vi "MagEncoder_cal_v3.vi"() -> ()   [LabVIEW 2014]
uses:
  <vilib>/rvi/FXPMathLib/FxpSinAndCos/subVIs/nifxpmath_SinAndCos_SimConfig.ctl
  <vilib>/rvi/Emulation/niFpgaGetClockAttributes.vi
  <vilib>/rvi/Emulation/niFpgaSctlEmulationGetInTimedLoop.vi
  <vilib>/rvi/Emulation/niFpgaEmulationReportErrorSimple.vi
  <vilib>/rvi/Emulation/niFpgaProcessEmulError.vi
  <vilib>/rvi/interface/RandomDataEmulation/nirviRandomDataMultiElementFPGAFIFO.vi
  <instcachedir>/0/nirviRandomDataMultiElementFPGAFIFO_AD0CFC12EF974623A9C2E4184BC062B2.lvgen/nirviRandomDataMultiElementFPGAFIFO_AD0CFC12EF974623A9C2E4184BC062B2_025.vi
  <vilib>/rvi/interface/RandomDataEmulation/niFpgaRandomDataHandleErrors.vi
  <vilib>/rvi/Emulation/niFpgaCriticalErrorInLSC.vi
  <vilib>/rvi/FXPMathLib/FxpSinAndCos/simVIs/DllFxpSinAndCosTemp_sub.vi
  <vilib>/rvi/eio/common/nirviEmuTemplateMethod_errors.vi
  <vilib>/rvi/DataTransferAndStorage/Container/XNode/niFpgaContainer.xnode
  <vilib>/rvi/interface/RandomDataEmulation/nirviRandomDataFpgaMultiElementTemplate.vi
  <vilib>/rvi/FXPMathLib/FxpSinAndCos/XNode/nifxpmath_SinAndCos.xnode
  <vilib>/eio/EIONode/EIONode.xnode
  <vilib>/rvi/Analysis/measure/butterworth/XNode/niFpgaButterworthFilter.xnode
panel:
  in  "Vy (mm/s)":fxp<+/-,30,6>
  out "Dyr_ramp":fxp<+/-,32,7>
  in  "Dyr_stroke":fxp<+/-,32,7>
  out "Dpr_ramp":fxp<+/-,32,7>
  in  "Dpr_stroke":fxp<+/-,32,7>
  in  "Vp (mm/s)":fxp<+/-,30,6>
  out "omega_p (Mavg w. f)":fxp<+/-,36,18>
  in  "scaled coefficients":i32[](array[numeric])=[946630756, 63555534]
  in  "FIFO":i16(ring) items=["Pitch_F+P", "Yaw_F+P"]
  out "PID (kHz)":fxp<+/-,20,10>
  out "Dy1_d (T)":fxp<+/-,36,13>
  out "omega_y1 (T)":fxp<+/-,36,13>
  out "Dp1_d (T)":fxp<+/-,36,13>
  out "omega_p1 (T)":fxp<+/-,36,13>
  out "Dy2_d (T)":fxp<+/-,36,13>
  out "Dp2_d (T)":fxp<+/-,36,13>
  out "omega_y2 (T)":fxp<+/-,36,13>
  out "omega_p2 (T)":fxp<+/-,36,13>
  out "mt_omega_y2":u32
  out "mt_omega_p2":u32
  out "rad_y2":fxp<+/-,33,20>
  out "D_y2":fxp<+/-,32,7>
  out "rad_y1":fxp<+/-,33,20>
  out "D_y1":fxp<+/-,32,7>
  out "Encoder Position_y1":i32
  out "Encoder Position_y2":i32
  out "Encoder Position_p2":i32
  out "D_p2":fxp<+/-,32,7>
  out "rad_p2":fxp<+/-,33,20>
  out "D_p1":fxp<+/-,32,7>
  out "rad_p1":fxp<+/-,33,20>
  out "Encoder Position_p1":i32
  in  "Mag. factor_y":fxp<+/-,20,3>
  in  "Mag. encoder_y":bool
  out "omega_y (rad/s)":fxp<+/-,36,13>
  out "Dy_d (mm/s)":fxp<+/-,36,13>
  in  "Vy. Est.":i16(ring) items=["T", "Mavg"]
  out "omega_y (Mavg)":fxp<+/-,36,14>
  out "Dy_d (Mavg)":fxp<+/-,36,14>
  in  "Dy_d_M_avg_Tc (uSec)":i32
  out "Dp_d (Mavg)":fxp<+/-,36,14>
  out "omega_p (Mavg)":fxp<+/-,36,14>
  in  "Dp_d_M_avg_Tc (uSec)":i32
  out "Dp_d (T)":fxp<+/-,36,13>
  out "omega_p (T)":fxp<+/-,36,13>
  in  "Vp. Est.":i16(ring) items=["T", "Mavg"]
  in  "Mag. factor_p":fxp<+/-,20,3>
  in  "Mag. encoder_p":bool
  in  "Belt_out_p":fxp<+/-,7,7>
  in  "Belt_in_p":fxp<+/-,6,6>
  in  "Belt_out_y":fxp<+/-,7,7>
  in  "Belt_in_y":fxp<+/-,6,6>
  in  "mt0_omega_p":u32
  in  "Encoder reset":bool
  out "Dpr_sin":fxp<+/-,32,7>
  in  "Sin offset_p":fxp<+/-,22,7>
  in  "Sin magnitude_p":fxp<+/-,21,6>
  in  "Sin wave freq._p (Hz)":fxp<+/-,32,6>
  in  "Dpr_step":fxp<+/-,32,7>
  out "Dpr_for":fxp<+/-,32,7>
  in  "Command_p":i16(ring) items=["Step", "Sine", "Ramp"]
  out "Fp_PID":fxp<+/-,36,16>
  in  "Kp_p":fxp<+/-,32,13>
  out "va_p":fxp<+/-,36,7>
  out "vb_p":fxp<+/-,37,8>
  out "vq_p_F":fxp<+/-,20,5> format="%.57g"
  out "vd_p_F":fxp<+/-,20,5>
  in  "Stop motor_p":bool
  out "Dp_d (mm/s)":fxp<+/-,36,13>
  out "omega_p (rad/s)":fxp<+/-,36,13>
  out "mt_omega_p1":u32
  out "rad_p(NrTheta)":fxp<+/-,33,20>
  out "D_p(mm)":fxp<+/-,32,7>
  out "Encoder Position_p":i32
  in  "Encoder reset_p":bool
  out "Dyr_for":fxp<+/-,32,7>
  in  "Command_y":i16(ring) items=["Step", "Sine", "Ramp"]
  out "vb_y":fxp<+/-,38,8>
  out "va_y":fxp<+/-,38,8>
  out "Dyr_sin":fxp<+/-,32,7>
  in  "Sin offset_y":fxp<+/-,22,7>
  in  "Sin magnitude_y":fxp<+/-,21,6>
  out "Time now(s)":fxp<+,52,14>
  in  "Sin wave freq._y (Hz)":fxp<+/-,32,6>
  in  "Dyr_step":fxp<+/-,32,7>
  out "Fy_PID":fxp<+/-,36,16>
  in  "Kp_y":fxp<+/-,32,13>
  out "vq_y_F":fxp<+/-,20,5> format="%.57g"
  out "vd_y_F":fxp<+/-,20,5>
  in  "Stop motor_y":bool
  out "Dy_d (T)":fxp<+/-,36,13>
  out "omega_y (T)":fxp<+/-,36,13>
  in  "mt0_omega_y":u32
  out "mt_omega_y1":u32
  out "rad_y(NrTheta)":fxp<+/-,33,20>
  out "D_y(mm)":fxp<+/-,32,7>
  out "Encoder Position_y":i32
  in  "Encoder reset_y":bool
  in  "Ini coe.":bool
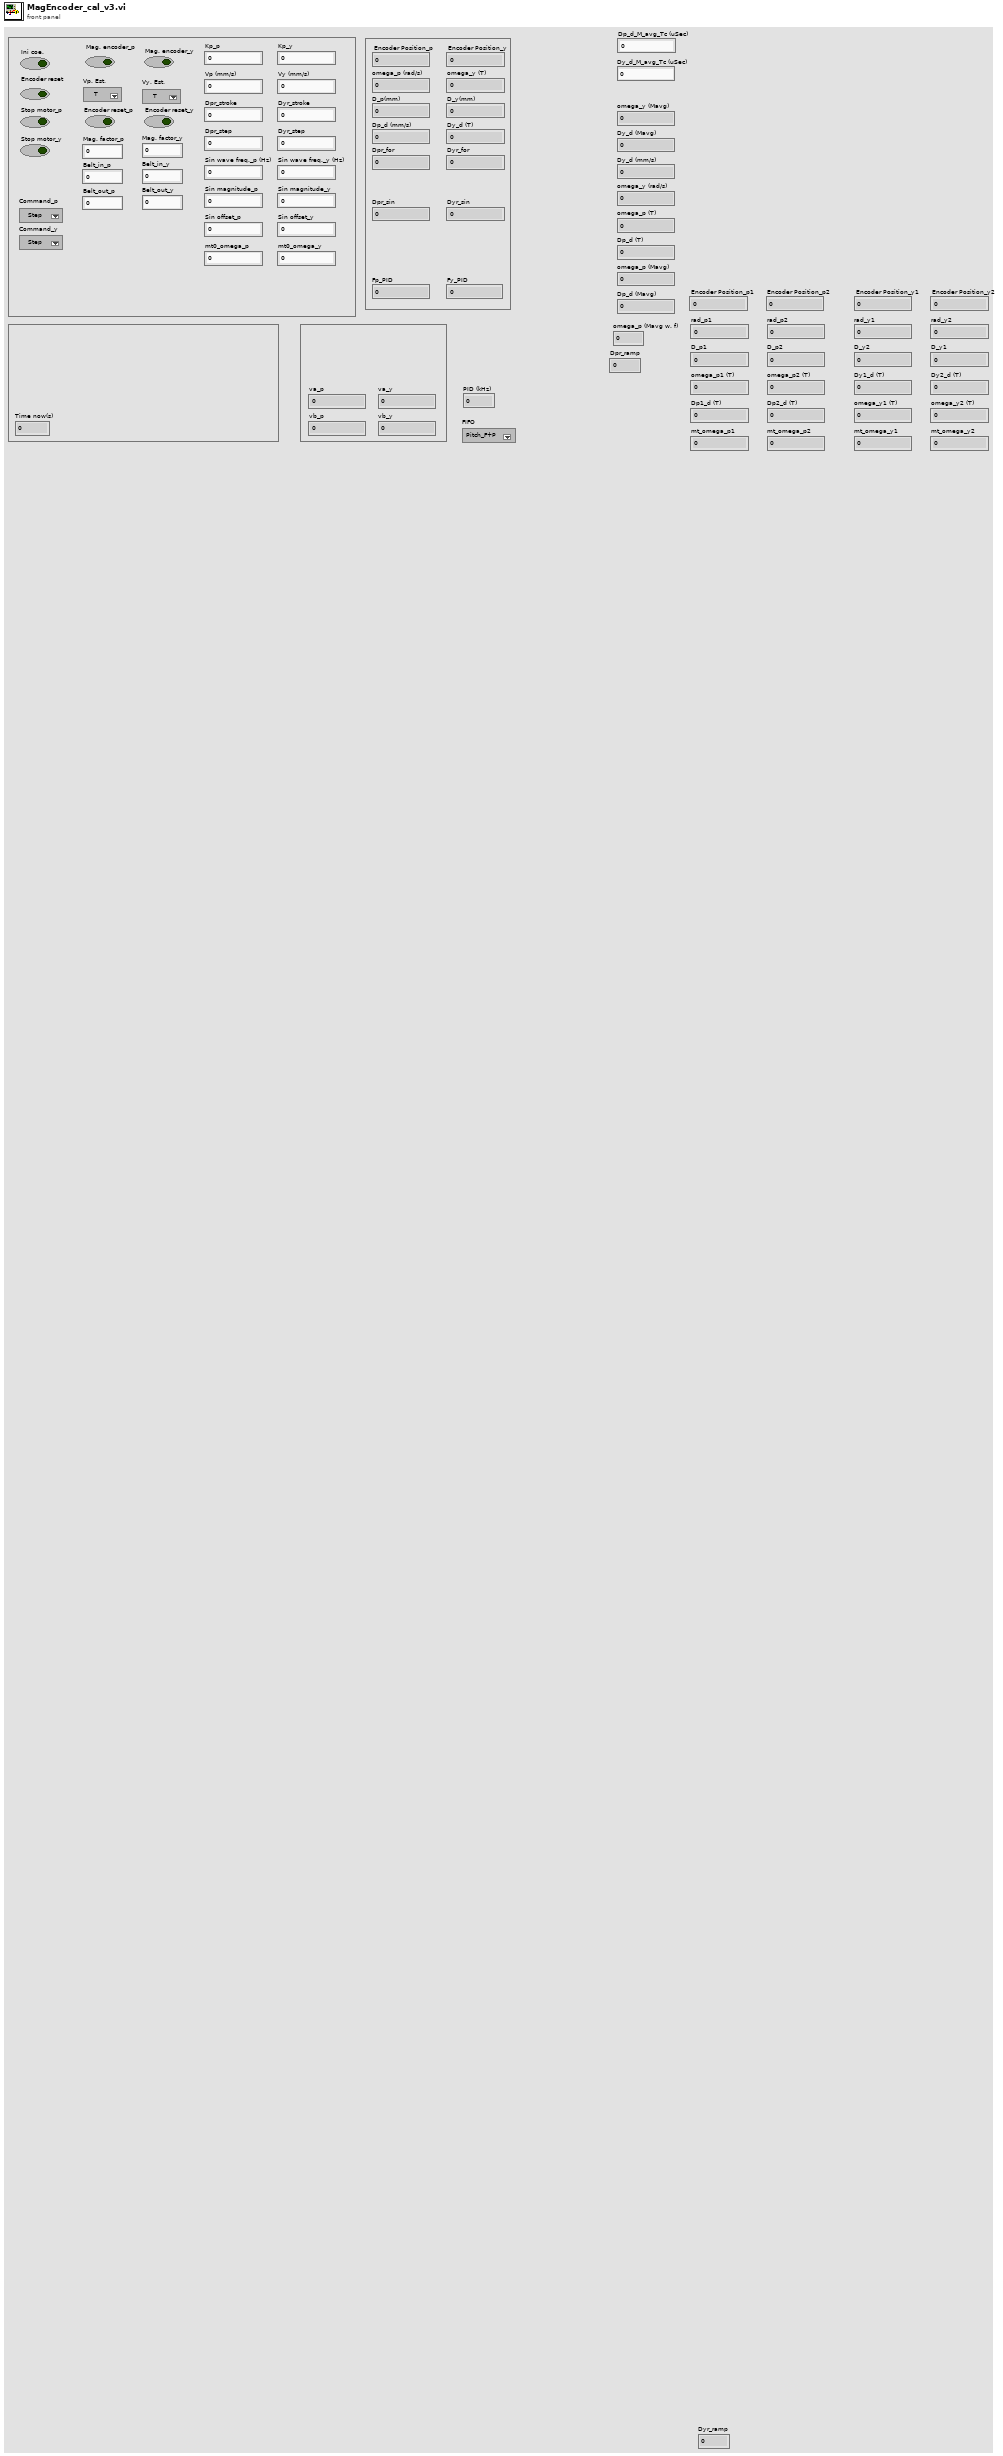
[diagram p1: front panel]
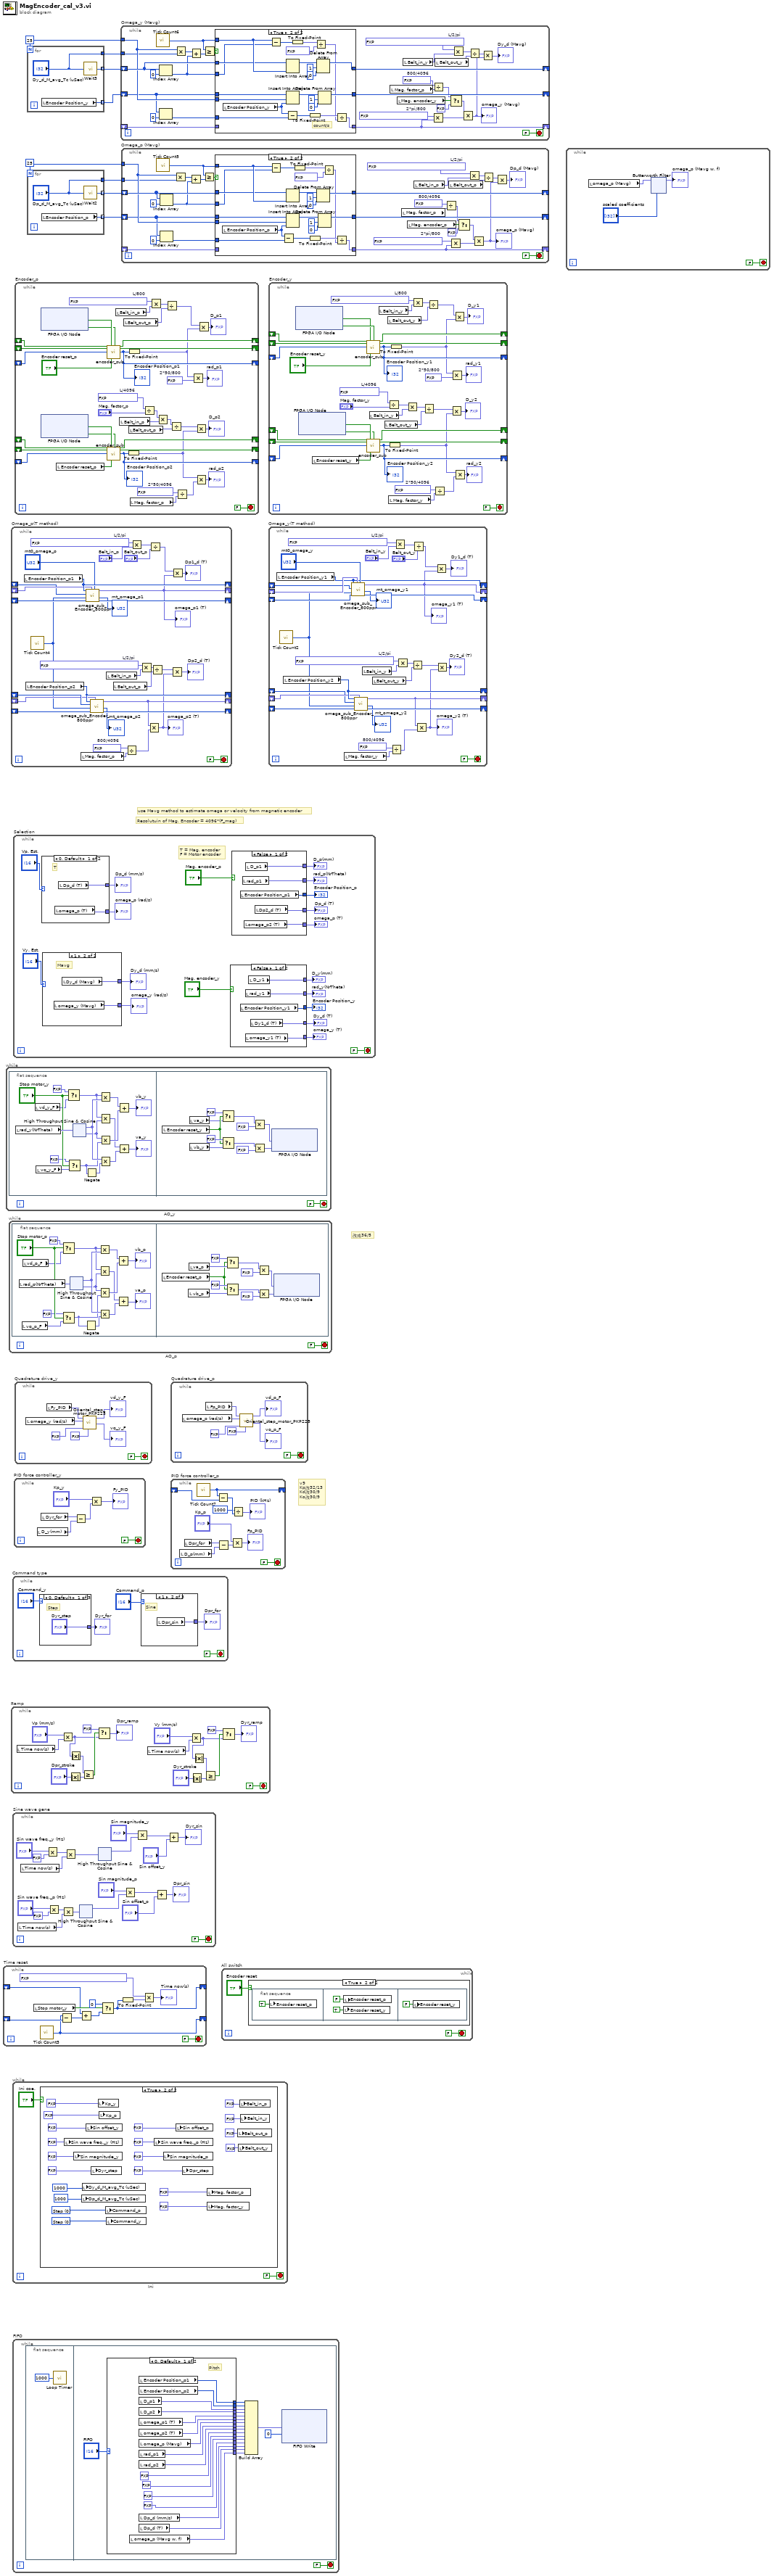
[diagram p0: block diagram]
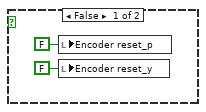
[diagram p4: hidden frame]
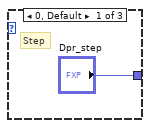
[diagram p5: hidden frame]
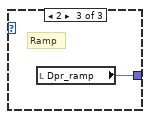
[diagram p6: hidden frame]
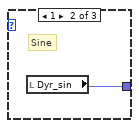
[diagram p7: hidden frame]
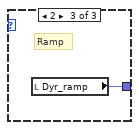
[diagram p8: hidden frame]
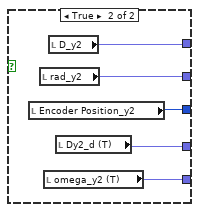
[diagram p9: hidden frame]
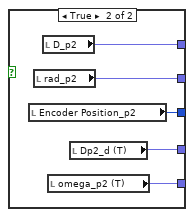
[diagram p10: hidden frame]
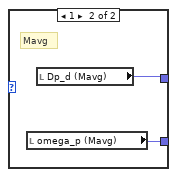
[diagram p11: hidden frame]
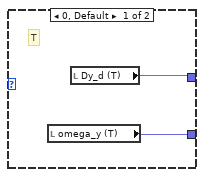
[diagram p12: hidden frame]
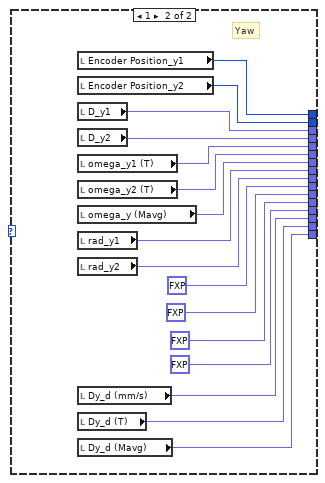
[diagram p14: hidden frame]
diagram:
  w5 = 25
  w8 = 25
  # "改成36/5"
  # "v9\nKp改32/13\nKd改30/9\nKo改30/9"
  # "Resolutuin of Mag. Encoder = 4096*(F_mag)"
  # "use Mavg method to estimate omega or velocity from magnetic encoder"
  n1 = while "Time reset" {
    shift-right: [w18] -> _
    shift-left: _ -> [w19]
    shift-right: [w13] -> _
    shift-left: _ -> [w14]
    stop <- FALSE stop-if-true
    n2 = local read "Stop motor_y"() -> (w20:bool)
    n3 = call "Tick Count3"() -> ("Tick Count(uSec)"=w18:u32)
    n4 = Subtract(x=w18, y=w19) -> (x-y=w17:u32)
    n5 = Add(x=w14, y=w17) -> (x+y=w16:u32)
    n6 = Select(t=u32 0, s=w20, f=w16) -> (s? t:f=w13:u32)
    n7 = To Fixed-Point(number=w13) -> (fixed-point=w12:fxp<+,32,32>)  [unwired: 1 in]
    n8 = Multiply(x=fxp<+,20,-18> 1.0000003385357559e-06, y=w12) -> (x*y=→"Time now(s)":fxp<+,52,14>)
  }
  n9 = while "AO_y" {
    stop <- FALSE stop-if-true
    n10 = flat-sequence {
      frame #0 {
        n11 = local read "rad_y(NrTheta)"() -> (w38:fxp<+/-,33,20>)
        n12 = local read "vd_y_F"() -> (w36:fxp<+/-,20,5>)
        n13 = local read "vq_y_F"() -> (w35:fxp<+/-,20,5>)
        n14 = Select(t=fxp<+/-,20,5> 0.0, s="Stop motor_y", f=w36) -> (s? t:f=w30:fxp<+/-,20,5>)
        n15 = Select(t=fxp<+/-,20,5> 0.0, s="Stop motor_y", f=w35) -> (s? t:f=w29:fxp<+/-,20,5>)
        n16 = xnode "High Throughput Sine & Cosine"("x (pi)"=w38) -> ("sin(x)"=w32:fxp<+/-,17,2>, "cos(x)"=w31:fxp<+/-,17,2>)
        n17 = Negate(x=w29) -> (-x=w28:fxp<+/-,21,6>)
        n18 = Multiply(x=w30, y=w32) -> (x*y=w27:fxp<+/-,37,7>)
        n19 = Multiply(x=w30, y=w31) -> (x*y=w25:fxp<+/-,37,7>)
        n20 = Multiply(x=w31, y=w29) -> (x*y=w26:fxp<+/-,37,7>)
        n21 = Multiply(x=w32, y=w28) -> (x*y=w24:fxp<+/-,36,6>)
        n22 = Add(x=w27, y=w26) -> (x+y=→"vb_y":fxp<+/-,38,8>)
        n23 = Add(x=w25, y=w24) -> (x+y=→"va_y":fxp<+/-,37,7>)
      }
      frame #1 {
        n24 = local read "Encoder reset_y"() -> (w71:bool)
        n25 = local read "va_y"() -> (w70:fxp<+/-,38,8>)
        n26 = local read "vb_y"() -> (w69:fxp<+/-,38,8>)
        n27 = Select(t=fxp<+,2,2> 3.0, s=w71, f=w70) -> (s? t:f=w75:fxp<+/-,38,8>)
        n28 = Select(t=fxp<+,1,1> 0.0, s=w71, f=w69) -> (s? t:f=w74:fxp<+/-,38,8>)
        n29 = Multiply(x=w75, y=fxp<+/-,1,0> -0.5) -> (x*y=w78:fxp<+/-,36,6>)
        n30 = Multiply(x=w74, y=fxp<+/-,1,0> -0.5) -> (x*y=w79:fxp<+/-,36,5>)
        n31 = xnode "FPGA I/O Node"("Mod8/AO2"=w78, "Mod8/AO3"=w79) -> ()  [unwired: 2 in, 2 out]
      }
    }
  }
  n32 = while "AO_p" {
    stop <- FALSE stop-if-true
    n33 = flat-sequence {
      frame #0 {
        n34 = local read "rad_p(NrTheta)"() -> (w92:fxp<+/-,33,20>)
        n35 = local read "vq_p_F"() -> (w93:fxp<+/-,20,5>)
        n36 = local read "vd_p_F"() -> (w95:fxp<+/-,20,5>)
        n37 = Select(t=fxp<+/-,20,5> 0.0, s="Stop motor_p", f=w95) -> (s? t:f=w84:fxp<+/-,20,5>)
        n38 = Select(t=fxp<+,1,1> 0.0, s="Stop motor_p", f=w93) -> (s? t:f=w83:fxp<+/-,20,5>)
        n39 = xnode "High Throughput Sine & Cosine"("x (pi)"=w92) -> ("sin(x)"=w86:fxp<+/-,16,2>, "cos(x)"=w85:fxp<+/-,16,2>)
        n40 = Negate(x=w83) -> (-x=w91:fxp<+/-,21,6>)
        n41 = Multiply(x=w84, y=w86) -> (x*y=w90:fxp<+/-,36,7>)
        n42 = Multiply(x=w84, y=w85) -> (x*y=w88:fxp<+/-,36,7>)
        n43 = Multiply(x=w85, y=w83) -> (x*y=w89:fxp<+/-,36,7>)
        n44 = Multiply(x=w86, y=w91) -> (x*y=w87:fxp<+/-,35,6>)
        n45 = Add(x=w90, y=w89) -> (x+y=→"vb_p":fxp<+/-,37,8>)
        n46 = Add(x=w88, y=w87) -> (x+y=→"va_p":fxp<+/-,36,7>)
      }
      frame #1 {
        n47 = local read "Encoder reset_p"() -> (w128:bool)
        n48 = local read "vb_p"() -> (w129:fxp<+/-,37,8>)
        n49 = local read "va_p"() -> (w130:fxp<+/-,36,7>)
        n50 = Select(t=fxp<+,2,2> 3.0, s=w128, f=w130) -> (s? t:f=w136:fxp<+/-,36,7>)
        n51 = Select(t=fxp<+,1,1> 0.0, s=w128, f=w129) -> (s? t:f=w135:fxp<+/-,37,8>)
        n52 = Multiply(x=w136, y=fxp<+/-,1,0> -0.5) -> (x*y=w131:fxp<+/-,36,5>)
        n53 = Multiply(x=w135, y=fxp<+/-,1,0> -0.5) -> (x*y=w132:fxp<+/-,36,5>)
        n54 = xnode "FPGA I/O Node"("Mod8/AO0"=w131, "Mod8/AO1"=w132) -> ()  [unwired: 2 in, 2 out]
      }
    }
  }
  n55 = while "Ramp" {
    stop <- FALSE stop-if-true
    n56 = local read "Time now(s)"() -> (w156:fxp<+,52,14>)
    n57 = Multiply(x="Vp (mm/s)", y=w156) -> (x*y=w143:fxp<+/-,64,20>)
    n58 = Absolute Value(x="Dpr_stroke") -> (abs(x)=w145:fxp<+,32,7>)
    n59 = Absolute Value(x=w143) -> (abs(x)=w144:fxp<+,64,20>)
    n60 = Greater Or Equal?(x=w144, y=w145) -> (x >= y?=w155:bool)
    n61 = Select(t=fxp<+/-,64,46> 0.0, s=w155, f=w143) -> (s? t:f=→"Dpr_ramp":fxp<+/-,64,46>)
    n62 = local read "Time now(s)"() -> (w149:fxp<+,52,14>)
    n63 = Multiply(x="Vy (mm/s)", y=w149) -> (x*y=w139:fxp<+/-,64,20>)
    n64 = Absolute Value(x="Dyr_stroke") -> (abs(x)=w141:fxp<+,32,7>)
    n65 = Absolute Value(x=w139) -> (abs(x)=w140:fxp<+,64,20>)
    n66 = Greater Or Equal?(x=w140, y=w141) -> (x >= y?=w152:bool)
    n67 = Select(t=fxp<+/-,64,46> 0.0, s=w152, f=w139) -> (s? t:f=→"Dyr_ramp":fxp<+/-,64,46>)
  }
  n68 = while "Omega_p(T method)" {
    shift-right: [w190] -> _
    shift-left: _ -> [w188]
    shift-right: [w161] -> _
    shift-left: _ -> [w189]
    shift-right: [w186] -> _
    shift-left: _ -> [w187]
    shift-right: [w177] -> _
    shift-left: _ -> [w176]
    shift-right: [w170] -> _
    shift-left: _ -> [w175]
    shift-right: [w174] -> _
    shift-left: _ -> [w173]
    stop <- FALSE stop-if-true
    w168 = fxp<+/-,32,0> 0.3183098859153688  # L/2/pi
    w179 = fxp<+,32,0> 0.1953125  # 800/4096
    w183 = fxp<+/-,32,0> 0.3183098859153688  # L/2/pi
    n69 = local read "Encoder Position_p1"() -> (w190:i32)
    n70 = local read "Encoder Position_p2"() -> (w177:i32)
    n71 = call "Tick Count4"() -> ("Tick Count(Ticks)"=w172:u32)
    n72 = local read "Mag. factor_p"() -> (w178:fxp<+/-,20,3>)
    n73 = call "omega_sub_Encoder_800ppr.vi"("mt0"="mt0_omega_p", "omega_pre"=w189, "ticks_m_pre"=w187, "ticks"=w172, "count_pre"=w188, "count"=w190) -> ("ticks_m"=w186:u32, "mt"=→"mt_omega_p1":u32, "omega"=w161:fxp<+/-,36,13>)  [unwired: 3 in]
    "omega_p1 (T)" <- w161
    n74 = call "omega_sub_Encoder_800ppr.vi"("omega_pre"=w175, "ticks_m_pre"=w173, "ticks"=w172, "count_pre"=w176, "count"=w177) -> ("ticks_m"=w174:u32, "mt"=→"mt_omega_p2":u32, "omega"=w170:fxp<+/-,36,13>)  [unwired: 4 in]
    n75 = local read "Belt_in_p"() -> (w166:fxp<+/-,6,6>)
    n76 = local read "Belt_out_p"() -> (w165:fxp<+/-,7,7>)
    n77 = Divide(x=w179, y=w178) -> (x/y=w169:fxp<+/-,32,1>)
    n78 = Multiply(x=w183, y="Belt_in_p") -> (x*y=w181:fxp<+/-,38,6>)
    n79 = Multiply(x=w168, y=w166) -> (x*y=w167:fxp<+/-,38,6>)
    n80 = Multiply(x=w170, y=w169) -> (x*y=w159:fxp<+/-,36,13>)
    "omega_p2 (T)" <- w159
    n81 = Divide(x=w181, y="Belt_out_p") -> (x/y=w162:fxp<+/-,20,1>)
    n82 = Divide(x=w167, y=w165) -> (x/y=w160:fxp<+/-,45,6>)
    n83 = Multiply(x=w160, y=w159) -> (x*y=→"Dp2_d (T)":fxp<+/-,36,13>)
    n84 = Multiply(x=w162, y=w161) -> (x*y=→"Dp1_d (T)":fxp<+/-,36,13>)
  }
  n85 = while "Command type" {
    stop <- FALSE stop-if-true
    n86 = case shown="0, Default" "Command_y" {
      tunnel: ["Dyr_step" w200 w201] -> w194
      frame 0, Default {
        # "Step"
      }
      frame 1 {
        # "Sine"
        n87 = local read "Dyr_sin"() -> (w200:fxp<+/-,32,7>)
      }
      frame 2 {
        # "Ramp"
        n88 = local read "Dyr_ramp"() -> (w201:fxp<+/-,32,7>)
      }
    }
    "Dyr_for" <- w194
    n89 = case shown="1" "Command_p" {
      tunnel: ["Dpr_step" w197 w198] -> w192
      frame 0, Default {
        # "Step"
      }
      frame 1 {
        # "Sine"
        n90 = local read "Dpr_sin"() -> (w197:fxp<+/-,32,7>)
      }
      frame 2 {
        # "Ramp"
        n91 = local read "Dpr_ramp"() -> (w198:fxp<+/-,32,7>)
      }
    }
    "Dpr_for" <- w192
  }
  n92 = while "Sine wave gene" {
    stop <- FALSE stop-if-true
    n93 = local read "Time now(s)"() -> (w208:fxp<+,52,14>)
    n94 = local read "Time now(s)"() -> (w219:fxp<+,52,14>)
    n95 = Multiply(x="Sin wave freq._y (Hz)", y=fxp<+/-,10,3> 2.0) -> (x*y=w220:fxp<+/-,41,9>)
    n96 = Multiply(x="Sin wave freq._p (Hz)", y=fxp<+/-,10,3> 2.0) -> (x*y=w212:fxp<+/-,42,9>)
    n97 = Multiply(x=w212, y=w208) -> (x*y=w209:fxp<+/-,41,19>)
    n98 = Multiply(x=w220, y=w219) -> (x*y=w218:fxp<+/-,41,19>)
    n99 = xnode "High Throughput Sine & Cosine"("x (pi)"=w209) -> ("sin(x)"=w203:fxp<+/-,20,2>)  [unwired: 1 out]
    n100 = xnode "High Throughput Sine & Cosine"("x (pi)"=w218) -> ("sin(x)"=w213:fxp<+/-,20,2>)  [unwired: 1 out]
    n101 = Multiply(x="Sin magnitude_p", y=w203) -> (x*y=w206:fxp<+/-,41,8>)
    n102 = Multiply(x="Sin magnitude_y", y=w213) -> (x*y=w216:fxp<+/-,41,8>)
    n103 = Add(x=w206, y="Sin offset_p") -> (x+y=→"Dpr_sin":fxp<+/-,41,8>)
    n104 = Add(x=w216, y="Sin offset_y") -> (x+y=→"Dyr_sin":fxp<+/-,41,8>)
  }
  n105 = while "Ini" {
    stop <- FALSE stop-if-true
    n106 = case shown="True" "Ini coe." {
      frame False {
      }
      frame True {
        w298 = i16 0 items=["Step", "Sine"] ("Command_p")
        w299 = i16 0 items=["Step", "Sine"] ("Command_y")
        n107 = local write "Sin wave freq._y (Hz)"(fxp<+/-,32,6> 1.0 ("Sin wave freq. (Hz)")) -> ()
        n108 = local write "Sin magnitude_y"(fxp<+/-,22,7> 5.0 ("Sin magnitude")) -> ()
        n109 = local write "Dp_d_M_avg_Tc (uSec)"(u32 1000 ("D_d_M_avg_Tc (uSec)")) -> ()
        n110 = local write "Dy_d_M_avg_Tc (uSec)"(1000 ("Dy_d_M_avg_Tc (uSec)")) -> ()
        n111 = local write "Sin offset_y"(fxp<+/-,38,9> 0.0 ("Sin offset")) -> ()
        n112 = local write "Dyr_step"(fxp<+/-,22,7> 0.0 ("Dr")) -> ()
        n113 = local write "Kp_y"(fxp<+/-,36,9> 30.0 ("Kp")) -> ()
        n114 = local write "Kp_p"(fxp<+/-,36,9> 30.0 ("Kp_p")) -> ()
        n115 = local write "Command_p"(w298) -> ()
        n116 = local write "Command_y"(w299) -> ()
        n117 = local write "Sin wave freq._p (Hz)"(fxp<+/-,32,6> 1.0 ("Sin wave freq._p (Hz)")) -> ()
        n118 = local write "Sin magnitude_p"(fxp<+/-,21,6> 5.0 ("Sin magnitude_p")) -> ()
        n119 = local write "Sin offset_p"(fxp<+/-,22,7> 0.0 ("Sin offset_p")) -> ()
        n120 = local write "Dpr_step"(fxp<+/-,22,7> 0.0 ("Dpr_step")) -> ()
        n121 = local write "Mag. factor_y"(fxp<+/-,36,9> 1.0 ("Kd_p")) -> ()
        n122 = local write "Mag. factor_p"(fxp<+/-,36,9> 1.0 ("Ki_p")) -> ()
        n123 = local write "Belt_out_p"(fxp<+/-,7,7> 22.0 ("Belt_op")) -> ()
        n124 = local write "Belt_out_y"(fxp<+/-,7,7> 22.0 ("Belt_oy")) -> ()
        n125 = local write "Belt_in_p"(fxp<+/-,6,6> 16.0 ("Belt_mp")) -> ()
        n126 = local write "Belt_in_y"(fxp<+/-,6,6> 16.0 ("Belt_my")) -> ()
      }
    }
  }
  n127 = while "FIFO" {
    stop <- FALSE stop-if-true
    n128 = flat-sequence {
      frame #0 {
        n129 = call "Loop Timer"("Count(uSec)"=u32 1000) -> ()  [unwired: 1 out]
      }
      frame #1 {
        n130 = case shown="0, Default" "FIFO" {
          tunnel: [w341 w357] -> w325
          tunnel: [w340 w356] -> w324
          tunnel: [w339 w355] -> w323
          tunnel: [w338 w354] -> w322
          tunnel: [w335 w351] -> w320
          tunnel: [w336 w352] -> w319
          tunnel: [w337 w353] -> w318
          tunnel: [w333 w346] -> w317
          tunnel: [fxp<+,1,1> 0.0 fxp<+,1,1> 0.0] -> w316
          tunnel: [fxp<+,1,1> 0.0 fxp<+,1,1> 0.0] -> w315
          tunnel: [fxp<+,1,1> 0.0 fxp<+,1,1> 0.0] -> w314
          tunnel: [fxp<+,1,1> 0.0 fxp<+,1,1> 0.0] -> w313
          tunnel: [w332 w349] -> w312
          tunnel: [w331 w348] -> w311
          tunnel: [w330 w347] -> w310
          tunnel: [w334 w350] -> w308
          frame 0, Default {
            # "Pitch"
            n131 = local read "omega_p (Mavg w. f)"() -> (w330:fxp<+/-,36,18>)
            n132 = local read "Encoder Position_p1"() -> (w341:i32)
            n133 = local read "Encoder Position_p2"() -> (w340:i32)
            n134 = local read "D_p1"() -> (w339:fxp<+/-,32,7>)
            n135 = local read "D_p2"() -> (w338:fxp<+/-,32,7>)
            n136 = local read "omega_p1 (T)"() -> (w337:fxp<+/-,36,13>)
            n137 = local read "omega_p2 (T)"() -> (w336:fxp<+/-,36,13>)
            n138 = local read "omega_p (Mavg)"() -> (w335:fxp<+/-,36,14>)
            n139 = local read "rad_p1"() -> (w334:fxp<+/-,33,20>)
            n140 = local read "rad_p2"() -> (w333:fxp<+/-,33,20>)
            n141 = local read "Dp_d (mm/s)"() -> (w332:fxp<+/-,36,13>)
            n142 = local read "Dp_d (T)"() -> (w331:fxp<+/-,36,13>)
          }
          frame 1 {
            # "Yaw"
            n143 = local read "Encoder Position_y1"() -> (w357:i32)
            n144 = local read "Encoder Position_y2"() -> (w356:i32)
            n145 = local read "D_y1"() -> (w355:fxp<+/-,32,7>)
            n146 = local read "D_y2"() -> (w354:fxp<+/-,32,7>)
            n147 = local read "omega_y1 (T)"() -> (w353:fxp<+/-,36,13>)
            n148 = local read "omega_y2 (T)"() -> (w352:fxp<+/-,36,13>)
            n149 = local read "omega_y (Mavg)"() -> (w351:fxp<+/-,36,14>)
            n150 = local read "rad_y1"() -> (w350:fxp<+/-,33,20>)
            n151 = local read "rad_y2"() -> (w346:fxp<+/-,33,20>)
            n152 = local read "Dy_d (mm/s)"() -> (w349:fxp<+/-,36,13>)
            n153 = local read "Dy_d (T)"() -> (w348:fxp<+/-,36,13>)
            n154 = local read "Dy_d (Mavg)"() -> (w347:fxp<+/-,36,14>)
          }
        }
        n155 = Build Array(w325, w324, w323, w322, w318, w319, w320, w308, w317, w316, w315, w314, w313, w312, w311, w310) -> (w309:fxp<+/-,57,32>[])
        n156 = xnode ("FIFO Write")("Element"=w309, "Timeout"=0) -> ()  [unwired: 1 in, 2 out]
      }
    }
  }
  n157 = while "Selection" {
    stop <- FALSE stop-if-true
    # "T = Mag. encoder\nF = Motor encoder"
    n158 = case shown="0, Default" "Vp. Est." {
      tunnel: [w398 w399] -> w372
      tunnel: [w397 w400] -> w373
      frame 0, Default {
        # "T"
        n159 = local read "omega_p (T)"() -> (w398:fxp<+/-,36,13>)
        n160 = local read "Dp_d (T)"() -> (w397:fxp<+/-,36,13>)
      }
      frame 1 {
        # "Mavg"
        n161 = local read "omega_p (Mavg)"() -> (w399:fxp<+/-,36,14>)
        n162 = local read "Dp_d (Mavg)"() -> (w400:fxp<+/-,36,14>)
      }
    }
    "Dp_d (mm/s)" <- w373
    "omega_p (rad/s)" <- w372
    n163 = case shown="1" "Vy. Est." {
      tunnel: [w402 w404] -> w375
      tunnel: [w401 w403] -> w376
      frame 0, Default {
        # "T"
        n164 = local read "omega_y (T)"() -> (w401:fxp<+/-,36,13>)
        n165 = local read "Dy_d (T)"() -> (w402:fxp<+/-,36,13>)
      }
      frame 1 {
        # "Mavg"
        n166 = local read "omega_y (Mavg)"() -> (w403:fxp<+/-,36,14>)
        n167 = local read "Dy_d (Mavg)"() -> (w404:fxp<+/-,36,14>)
      }
    }
    "Dy_d (mm/s)" <- w375
    "omega_y (rad/s)" <- w376
    n168 = case shown="False" "Mag. encoder_y" {
      tunnel: [w381 w385] -> w363
      tunnel: [w380 w386] -> w364
      tunnel: [w379 w384] -> w366
      tunnel: [w377 w383] -> w360
      tunnel: [w378 w382] -> w359
      frame False {
        n169 = local read "Encoder Position_y1"() -> (w379:i32)
        n170 = local read "rad_y1"() -> (w381:fxp<+/-,33,20>)
        n171 = local read "omega_y1 (T)"() -> (w377:fxp<+/-,36,13>)
        n172 = local read "D_y1"() -> (w380:fxp<+/-,32,7>)
        n173 = local read "Dy1_d (T)"() -> (w378:fxp<+/-,36,13>)
      }
      frame True {
        n174 = local read "Encoder Position_y2"() -> (w384:i32)
        n175 = local read "rad_y2"() -> (w385:fxp<+/-,33,20>)
        n176 = local read "omega_y2 (T)"() -> (w383:fxp<+/-,36,13>)
        n177 = local read "D_y2"() -> (w386:fxp<+/-,32,7>)
        n178 = local read "Dy2_d (T)"() -> (w382:fxp<+/-,36,13>)
      }
    }
    "D_y(mm)" <- w364
    "rad_y(NrTheta)" <- w363
    "Encoder Position_y" <- w366
    "Dy_d (T)" <- w359
    "omega_y (T)" <- w360
    n179 = case shown="False" "Mag. encoder_p" {
      tunnel: [w391 w396] -> w368
      tunnel: [w390 w395] -> w369
      tunnel: [w389 w394] -> w370
      tunnel: [w387 w393] -> w362
      tunnel: [w388 w392] -> w361
      frame False {
        n180 = local read "Encoder Position_p1"() -> (w389:i32)
        n181 = local read "rad_p1"() -> (w390:fxp<+/-,33,20>)
        n182 = local read "omega_p2 (T)"() -> (w387:fxp<+/-,36,13>)
        n183 = local read "D_p1"() -> (w391:fxp<+/-,32,7>)
        n184 = local read "Dp2_d (T)"() -> (w388:fxp<+/-,36,13>)
      }
      frame True {
        n185 = local read "Encoder Position_p2"() -> (w394:i32)
        n186 = local read "rad_p2"() -> (w395:fxp<+/-,33,20>)
        n187 = local read "D_p2"() -> (w396:fxp<+/-,32,7>)
        n188 = local read "omega_p2 (T)"() -> (w393:fxp<+/-,36,13>)
        n189 = local read "Dp2_d (T)"() -> (w392:fxp<+/-,36,13>)
      }
    }
    "D_p(mm)" <- w368
    "rad_p(NrTheta)" <- w369
    "Encoder Position_p" <- w370
    "Dp_d (T)" <- w361
    "omega_p (T)" <- w362
  }
  n190 = while "PID force controller_y" {
    stop <- FALSE stop-if-true
    n191 = local read "D_y(mm)"() -> (w408:fxp<+/-,32,7>)
    n192 = local read "Dyr_for"() -> (w409:fxp<+/-,32,7>)
    n193 = Subtract(x=w409, y=w408) -> (x-y=w407:fxp<+/-,33,8>)
    n194 = Multiply(x="Kp_y", y=w407) -> (x*y=→"Fy_PID":fxp<+/-,64,20>)
  }
  n195 = while "Quadrature drive_y" {
    stop <- FALSE stop-if-true
    n196 = local read "omega_y (rad/s)"() -> (w417:fxp<+/-,36,13>)
    n197 = local read "Fy_PID"() -> (w413:fxp<+/-,36,16>)
    n198 = call "Oriental_step_motor_PKP225.vi"("F_Threshold"=fxp<+,12,12> 10.0, "dFmr"=fxp<+/-,25,15> 0.0, "omega"=w417, "Fmr"=w413) -> ("vq_F"=→"vq_y_F":fxp<+/-,20,5>, "vd_F"=→"vd_y_F":fxp<+/-,20,5>)  [unwired: 6 in]
  }
  n199 = while "Encoder_p" {
    shift-right: [w455] -> _
    shift-left: _ -> [w454]
    shift-right: [w456] -> _
    shift-left: _ -> [w453]
    shift-right: [w450] -> _
    shift-left: _ -> [w452]
    shift-right: [w441] -> _
    shift-left: _ -> [w440]
    shift-right: [w442] -> _
    shift-left: _ -> [w443]
    shift-right: [w437] -> _
    shift-left: _ -> [w438]
    stop <- FALSE stop-if-true
    w433 = fxp<+/-,20,-5> 0.00048828125  # L/4096
    w431 = fxp<+/-,16,1> 0.0244140625  # 2*50/4096
    w449 = fxp<+/-,20,-5> 0.002499997615814209  # L/800
    w423 = fxp<+/-,16,1> 0.125  # 2*50/800
    n200 = xnode "FPGA I/O Node"() -> ("Mod7/DIO0"=w458:bool, "Mod7/DIO1"=w457:bool)  [unwired: 2 in, 2 out]
    n201 = xnode "FPGA I/O Node"() -> ("Mod7/DIO4"=w445:bool, "Mod7/DIO5"=w444:bool)  [unwired: 2 in, 2 out]
    n202 = local read "Encoder reset_p"() -> (w439:bool)
    n203 = call "encoder_sub.vi"("A_pre"=w454, "B_pre"=w453, "Encoder Position_pre"=w452, "A input"=w458, "Encoder Position Reset"="Encoder reset_p", "B input"=w457) -> ("A"=w455:bool, "B"=w456:bool, "Encoder Position (Counts)"=w450:i32)  [unwired: 19 in]
    "Encoder Position_p1" <- w450
    n204 = call "encoder_sub.vi"("A_pre"=w440, "B_pre"=w443, "Encoder Position_pre"=w438, "A input"=w445, "Encoder Position Reset"=w439, "B input"=w444) -> ("A"=w441:bool, "B"=w442:bool, "Encoder Position (Counts)"=w437:i32)  [unwired: 19 in]
    "Encoder Position_p2" <- w437
    n205 = local read "Belt_in_p"() -> (w448:fxp<+/-,6,6>)
    n206 = local read "Belt_in_p"() -> (w434:fxp<+/-,6,6>)
    n207 = local read "Belt_out_p"() -> (w446:fxp<+/-,7,7>)
    n208 = To Fixed-Point(number=w437) -> (fixed-point=w419:fxp<+/-,32,32>)  [unwired: 1 in]
    n209 = To Fixed-Point(number=w450) -> (fixed-point=w424:fxp<+/-,32,32>)  [unwired: 1 in]
    n210 = local read "Belt_out_p"() -> (w436:fxp<+/-,7,7>)
    n211 = local read "Mag. factor_p"() -> (w430:fxp<+/-,20,3>)
    n212 = Divide(x=w433, y="Mag. factor_p") -> (x/y=w432:fxp<+/-,41,13>)
    n213 = Multiply(x=w449, y=w448) -> (x*y=w447:fxp<+/-,26,1>)
    n214 = Multiply(x=w432, y=w434) -> (x*y=w435:fxp<+/-,46,18>)
    n215 = Divide(x=w447, y=w446) -> (x/y=w426:fxp<+/-,33,1>)
    n216 = Divide(x=w435, y=w436) -> (x/y=w421:fxp<+/-,53,18>)
    n217 = Divide(x=w431, y=w430) -> (x/y=w418:fxp<+/-,32,1>)
    n218 = Multiply(x=w424, y=w423) -> (x*y=→"rad_p1":fxp<+/-,33,20>)
    n219 = Multiply(x=w421, y=w419) -> (x*y=→"D_p2":fxp<+/-,37,7>)
    n220 = Multiply(x=w419, y=w418) -> (x*y=→"rad_p2":fxp<+/-,33,20>)
    n221 = Multiply(x=w426, y=w424) -> (x*y=→"D_p1":fxp<+/-,32,7>)
  }
  n222 = for {
    N: w5 -> [_]
    tunnel: [w461] -> w4 mode=indexing
    tunnel: [w460] -> w3 mode=indexing
    tunnel: ["Dy_d_M_avg_Tc (uSec)"] -> w2
    n223 = local read "Encoder Position_y"() -> (w460:i32)
    n224 = call "Wait3"("Count(uSec)"="Dy_d_M_avg_Tc (uSec)") -> ("Tick Count(uSec)"=w461:u32)
  }
  n225 = for {
    N: w8 -> [_]
    tunnel: ["Dp_d_M_avg_Tc (uSec)"] -> w1
    tunnel: [w463] -> w7 mode=indexing
    tunnel: [w462] -> w6 mode=indexing
    n226 = local read "Encoder Position_p"() -> (w462:i32)
    n227 = call "Wait2"("Count(uSec)"="Dp_d_M_avg_Tc (uSec)") -> ("Tick Count(uSec)"=w463:u32)
  }
  n228 = while "Omega_y (Mavg)" {
    tunnel: w5 -> [w488]
    shift-right: [w486] -> _
    shift-left: w4 -> [w491]
    shift-right: [w485] -> _
    shift-left: w3 -> [w487]
    shift-right: [w480] -> _
    shift-left: _ -> [w484]
    tunnel: w2 -> [w479]
    stop <- FALSE stop-if-true
    w467 = fxp<+/-,32,0> 0.3183098859153688  # L/2/pi
    w476 = fxp<+,32,0> 0.1953125  # 800/4096
    w482 = fxp<+/-,27,3> 0.007853984832763672  # 2*pi/800
    n229 = call "Tick Count6"() -> ("Tick Count(uSec)"=w492:u32)
    n230 = Index Array(array=w491, index=0) -> (element=w490:u32)
    n231 = Index Array(array=w487, index=0) -> (element=w489:i32)
    n232 = Multiply(x=w488, y=w479) -> (x*y=w494:i32)
    n233 = Add(x=w494, y=w490) -> (x+y=w493:u32)
    n234 = Greater Or Equal?(x=w492, y=w493) -> (x >= y?=w483:bool)
    n235 = case shown="True" w483 {
      tunnel: w492 -> [_ w515]
      tunnel: w488 -> [_ w512]
      tunnel: w491 -> [w499 w514]
      tunnel: w490 -> [_ w513]
      tunnel: w489 -> [_ w509]
      tunnel: w487 -> [w498 w511]
      tunnel: [w497 w507] -> w480
      tunnel: [w499 w506] -> w486
      tunnel: [w498 w505] -> w485
      tunnel: w484 -> [w497 _]
      frame False {
      }
      frame True {
        # "count/s"
        n236 = local read "Encoder Position_y"() -> (w508:i32)
        n237 = Subtract(x=w515, y=w513) -> (x-y=w516:u32)
        n238 = Insert Into Array(array=w514, new element=w515) -> (w518:u32[])  [unwired: 1 in]
        n239 = Subtract(x=w508, y=w509) -> (x-y=w503:i32)
        n240 = Insert Into Array(array=w511, index=w512, new element=w508) -> (w519:i32[])
        n241 = To Fixed-Point(number=w516) -> (fixed-point=w502:fxp<+,32,32>)  [unwired: 1 in]
        n242 = To Fixed-Point(number=w503) -> (fixed-point=w510:fxp<+/-,32,32>)  [unwired: 1 in]
        n243 = Divide(x=w502, y=fxp<+,32,32> 1000000.0) -> (x/y=w501:fxp<+/-,64,32>)
        n244 = Delete From Array(array=w518, length=1, index=0) -> (array with subset deleted=w506:u32[])  [unwired: 1 out]
        n245 = Delete From Array(array=w519, length=1, index=0) -> (array with subset deleted=w505:i32[])  [unwired: 1 out]
        n246 = Divide(x=w510, y=w501) -> (x/y=w507:fxp<+/-,40,20>)
      }
    }
    n247 = local read "Mag. factor_p"() -> (w475:fxp<+/-,20,3>)
    n248 = local read "Mag. encoder_y"() -> (w478:bool)
    n249 = local read "Belt_in_y"() -> (w469:fxp<+/-,6,6>)
    n250 = Multiply(x=w482, y=w480) -> (x*y=w472:fxp<+/-,64,23>)
    n251 = Divide(x=w476, y=w475) -> (x/y=w474:fxp<+/-,32,1>)
    n252 = local read "Belt_out_y"() -> (w470:fxp<+/-,7,7>)
    n253 = Select(t=w474, s=w478, f=fxp<+/-,2,2> 1.0) -> (s? t:f=w473:fxp<+/-,33,2>)
    n254 = Multiply(x=w467, y=w469) -> (x*y=w468:fxp<+/-,38,6>)
    n255 = Multiply(x=w473, y=w472) -> (x*y=w471:fxp<+/-,64,25>)
    "omega_y (Mavg)" <- w471
    n256 = Divide(x=w468, y=w470) -> (x/y=w466:fxp<+/-,45,6>)
    n257 = Multiply(x=w466, y=w471) -> (x*y=→"Dy_d (Mavg)":fxp<+/-,64,30>)
  }
  n258 = while "Omega_p (Mavg)" {
    tunnel: w8 -> [w545]
    shift-right: [w543] -> _
    shift-left: w7 -> [w548]
    shift-right: [w542] -> _
    shift-left: w6 -> [w544]
    shift-right: [w541] -> _
    shift-left: _ -> [w540]
    tunnel: w1 -> [w538]
    stop <- FALSE stop-if-true
    w527 = fxp<+/-,27,3> 0.007853984832763672  # 2*pi/800
    w529 = fxp<+,32,0> 0.1953125  # 800/4096
    w526 = fxp<+/-,32,0> 0.3183098859153688  # L/2/pi
    n259 = call "Tick Count5"() -> ("Tick Count(uSec)"=w549:u32)
    n260 = Index Array(array=w548, index=0) -> (element=w547:u32)
    n261 = Index Array(array=w544, index=0) -> (element=w546:i32)
    n262 = Multiply(x=w545, y=w538) -> (x*y=w551:i32)
    n263 = Add(x=w551, y=w547) -> (x+y=w550:u32)
    n264 = Greater Or Equal?(x=w549, y=w550) -> (x >= y?=w539:bool)
    n265 = case shown="True" w539 {
      tunnel: w549 -> [_ w572]
      tunnel: w545 -> [_ w569]
      tunnel: w548 -> [w556 w571]
      tunnel: w547 -> [_ w570]
      tunnel: w546 -> [_ w566]
      tunnel: w544 -> [w555 w568]
      tunnel: [w554 w564] -> w541
      tunnel: [w556 w563] -> w543
      tunnel: [w555 w562] -> w542
      tunnel: w540 -> [w554 _]
      frame False {
      }
      frame True {
        n266 = local read "Encoder Position_p"() -> (w565:i32)
        n267 = Subtract(x=w572, y=w570) -> (x-y=w573:u32)
        n268 = Subtract(x=w565, y=w566) -> (x-y=w557:i32)
        n269 = Insert Into Array(array=w571, new element=w572) -> (w575:u32[])  [unwired: 1 in]
        n270 = Insert Into Array(array=w568, index=w569, new element=w565) -> (w576:i32[])
        n271 = To Fixed-Point(number=w573) -> (fixed-point=w559:fxp<+,32,32>)  [unwired: 1 in]
        n272 = To Fixed-Point(number=w557) -> (fixed-point=w567:fxp<+/-,32,32>)  [unwired: 1 in]
        n273 = Delete From Array(array=w575, length=1, index=0) -> (array with subset deleted=w563:u32[])  [unwired: 1 out]
        n274 = Delete From Array(array=w576, length=1, index=0) -> (array with subset deleted=w562:i32[])  [unwired: 1 out]
        n275 = Divide(x=w559, y=fxp<+,32,32> 1000000.0) -> (x/y=w560:fxp<+/-,64,32>)
        n276 = Divide(x=w567, y=w560) -> (x/y=w564:fxp<+/-,40,20>)
      }
    }
    n277 = local read "Mag. factor_p"() -> (w530:fxp<+/-,20,3>)
    n278 = local read "Mag. encoder_p"() -> (w537:bool)
    n279 = local read "Belt_in_p"() -> (w534:fxp<+/-,6,6>)
    n280 = Divide(x=w529, y=w530) -> (x/y=w528:fxp<+/-,32,1>)
    n281 = local read "Belt_out_p"() -> (w533:fxp<+/-,7,7>)
    n282 = Multiply(x=w527, y=w541) -> (x*y=w535:fxp<+/-,64,23>)
    n283 = Select(t=w528, s=w537, f=fxp<+/-,2,2> 1.0) -> (s? t:f=w522:fxp<+/-,33,2>)
    n284 = Multiply(x=w526, y=w534) -> (x*y=w532:fxp<+/-,38,6>)
    n285 = Multiply(x=w522, y=w535) -> (x*y=w525:fxp<+/-,64,25>)
    "omega_p (Mavg)" <- w525
    n286 = Divide(x=w532, y=w533) -> (x/y=w524:fxp<+/-,45,6>)
    n287 = Multiply(x=w524, y=w525) -> (x*y=→"Dp_d (Mavg)":fxp<+/-,64,30>)
  }
  n288 = while "Quadrature drive_p" {
    stop <- FALSE stop-if-true
    n289 = local read "omega_p (rad/s)"() -> (w585:fxp<+/-,36,13>)
    n290 = local read "Fp_PID"() -> (w581:fxp<+/-,36,16>)
    n291 = call "Oriental_step_motor_PKP225.vi"("F_Threshold"=fxp<+,12,12> 10.0, "dFmr"=fxp<+/-,25,15> 0.0, "omega"=w585, "Fmr"=w581) -> ("vq_F"=→"vq_p_F":fxp<+/-,20,5>, "vd_F"=→"vd_p_F":fxp<+/-,20,5>)  [unwired: 6 in]
  }
  n292 = while "PID force controller_p" {
    shift-right: [w596] -> _
    shift-left: _ -> [w595]
    stop <- FALSE stop-if-true
    n293 = local read "D_p(mm)"() -> (w590:fxp<+/-,32,7>)
    n294 = local read "Dpr_for"() -> (w591:fxp<+/-,32,7>)
    n295 = call "Tick Count7"() -> ("Tick Count(uSec)"=w596:u32)
    n296 = Subtract(x=w596, y=w595) -> (x-y=w594:u32)
    n297 = Subtract(x=w591, y=w590) -> (x-y=w589:fxp<+/-,33,8>)
    n298 = Multiply(x="Kp_p", y=w589) -> (x*y=→"Fp_PID":fxp<+/-,64,20>)
    n299 = Divide(x=u32 1000, y=w594) -> (x/y=→"PID (kHz)":fxp<+/-,20,7>)
  }
  n300 = while "All switch" {
    stop <- FALSE stop-if-true
    n301 = case shown="True" "Encoder reset" {
      frame False {
        n302 = local write "Encoder reset_p"(FALSE ("Encoder reset_p")) -> ()
        n303 = local write "Encoder reset_y"(FALSE ("Encoder reset_y")) -> ()
      }
      frame True {
        n304 = flat-sequence {
          frame #0 {
            n305 = local write "Encoder reset_p"(TRUE ("Encoder reset_p")) -> ()
          }
          frame #1 {
            n306 = local write "Encoder reset_y"(TRUE ("Encoder reset_y")) -> ()
            n307 = local write "Encoder reset_p"(FALSE ("Encoder reset_p")) -> ()
          }
          frame #2 {
            n308 = local write "Encoder reset_y"(FALSE ("Encoder reset_y")) -> ()
          }
        }
      }
    }
  }
  n309 = while "Omega_y(T method)" {
    shift-right: [w631] -> _
    shift-left: _ -> [w632]
    shift-right: [w608] -> _
    shift-left: _ -> [w634]
    shift-right: [w636] -> _
    shift-left: _ -> [w637]
    shift-right: [w624] -> _
    shift-left: _ -> [w622]
    shift-right: [w617] -> _
    shift-left: _ -> [w623]
    shift-right: [w620] -> _
    shift-left: _ -> [w621]
    stop <- FALSE stop-if-true
    w615 = fxp<+/-,32,0> 0.3183098859153688  # L/2/pi
    w626 = fxp<+,32,0> 0.1953125  # 800/4096
    w630 = fxp<+/-,32,0> 0.3183098859153688  # L/2/pi
    n310 = local read "Encoder Position_y1"() -> (w631:i32)
    n311 = call "Tick Count2"() -> ("Tick Count(Ticks)"=w618:u32)
    n312 = local read "Encoder Position_y2"() -> (w624:i32)
    n313 = local read "Mag. factor_y"() -> (w625:fxp<+/-,20,3>)
    n314 = call "omega_sub_Encoder_800ppr.vi"("mt0"="mt0_omega_y", "omega_pre"=w634, "ticks_m_pre"=w637, "ticks"=w618, "count_pre"=w632, "count"=w631) -> ("ticks_m"=w636:u32, "mt"=→"mt_omega_y1":u32, "omega"=w608:fxp<+/-,36,13>)  [unwired: 3 in]
    "omega_y1 (T)" <- w608
    n315 = call "omega_sub_Encoder_800ppr.vi"("omega_pre"=w623, "ticks_m_pre"=w621, "ticks"=w618, "count_pre"=w622, "count"=w624) -> ("ticks_m"=w620:u32, "mt"=→"mt_omega_y2":u32, "omega"=w617:fxp<+/-,36,13>)  [unwired: 4 in]
    n316 = local read "Belt_in_y"() -> (w614:fxp<+/-,6,6>)
    n317 = local read "Belt_out_y"() -> (w612:fxp<+/-,7,7>)
    n318 = Divide(x=w626, y=w625) -> (x/y=w616:fxp<+/-,32,1>)
    n319 = Multiply(x=w630, y="Belt_in_y") -> (x*y=w628:fxp<+/-,38,6>)
    n320 = Multiply(x=w615, y=w614) -> (x*y=w613:fxp<+/-,38,6>)
    n321 = Divide(x=w613, y=w612) -> (x/y=w606:fxp<+/-,45,6>)
    n322 = Divide(x=w628, y="Belt_out_y") -> (x/y=w609:fxp<+/-,20,1>)
    n323 = Multiply(x=w617, y=w616) -> (x*y=w605:fxp<+/-,36,13>)
    "omega_y2 (T)" <- w605
    n324 = Multiply(x=w609, y=w608) -> (x*y=→"Dy1_d (T)":fxp<+/-,36,13>)
    n325 = Multiply(x=w606, y=w605) -> (x*y=→"Dy2_d (T)":fxp<+/-,36,13>)
  }
  n326 = while "Encoder_y" {
    shift-right: [w676] -> _
    shift-left: _ -> [w668]
    shift-right: [w675] -> _
    shift-left: _ -> [w667]
    shift-right: [w666] -> _
    shift-left: _ -> [w664]
    shift-right: [w672] -> _
    shift-left: _ -> [w669]
    shift-right: [w671] -> _
    shift-left: _ -> [w670]
    shift-right: [w665] -> _
    shift-left: _ -> [w663]
    stop <- FALSE stop-if-true
    w653 = fxp<+/-,16,1> 0.0244140625  # 2*50/4096
    w658 = fxp<+/-,20,-5> 0.00048828125  # L/4096
    w661 = fxp<+/-,20,-5> 0.002499997615814209  # L/800
    w643 = fxp<+/-,16,1> 0.125  # 2*50/800
    n327 = xnode "FPGA I/O Node"() -> ("Mod7/DIO2"=w677:bool, "Mod7/DIO3"=w678:bool)  [unwired: 2 in, 2 out]
    n328 = xnode "FPGA I/O Node"() -> ("Mod7/DIO6"=w674:bool, "Mod7/DIO7"=w673:bool)  [unwired: 2 in, 2 out]
    n329 = local read "Encoder reset_y"() -> (w648:bool)
    n330 = call "encoder_sub.vi"("A_pre"=w668, "B_pre"=w667, "Encoder Position_pre"=w664, "A input"=w677, "Encoder Position Reset"="Encoder reset_y", "B input"=w678) -> ("A"=w676:bool, "B"=w675:bool, "Encoder Position (Counts)"=w666:i32)  [unwired: 19 in]
    "Encoder Position_y1" <- w666
    n331 = call "encoder_sub.vi"("A_pre"=w669, "B_pre"=w670, "Encoder Position_pre"=w663, "A input"=w674, "Encoder Position Reset"=w648, "B input"=w673) -> ("A"=w672:bool, "B"=w671:bool, "Encoder Position (Counts)"=w665:i32)  [unwired: 19 in]
    "Encoder Position_y2" <- w665
    n332 = local read "Belt_in_y"() -> (w656:fxp<+/-,6,6>)
    n333 = local read "Belt_in_y"() -> (w660:fxp<+/-,6,6>)
    n334 = local read "Belt_out_y"() -> (w654:fxp<+/-,7,7>)
    n335 = Divide(x=w658, y="Mag. factor_y") -> (x/y=w657:fxp<+/-,41,13>)
    n336 = local read "Belt_out_y"() -> (w659:fxp<+/-,7,7>)
    n337 = To Fixed-Point(number=w665) -> (fixed-point=w640:fxp<+/-,32,32>)  [unwired: 1 in]
    n338 = local read "Mag. factor_y"() -> (w652:fxp<+/-,20,3>)
    n339 = To Fixed-Point(number=w666) -> (fixed-point=w644:fxp<+/-,32,32>)  [unwired: 1 in]
    n340 = Multiply(x=w657, y=w656) -> (x*y=w655:fxp<+/-,46,18>)
    n341 = Multiply(x=w661, y=w660) -> (x*y=w662:fxp<+/-,26,1>)
    n342 = Divide(x=w655, y=w654) -> (x/y=w642:fxp<+/-,53,18>)
    n343 = Divide(x=w662, y=w659) -> (x/y=w646:fxp<+/-,33,1>)
    n344 = Divide(x=w653, y=w652) -> (x/y=w639:fxp<+/-,32,1>)
    n345 = Multiply(x=w642, y=w640) -> (x*y=→"D_y2":fxp<+/-,37,7>)
    n346 = Multiply(x=w644, y=w643) -> (x*y=→"rad_y1":fxp<+/-,33,20>)
    n347 = Multiply(x=w646, y=w644) -> (x*y=→"D_y1":fxp<+/-,32,7>)
    n348 = Multiply(x=w640, y=w639) -> (x*y=→"rad_y2":fxp<+/-,33,20>)
  }
  n349 = while {
    stop <- FALSE stop-if-true
    n350 = local read "omega_p (Mavg)"() -> (w682:fxp<+/-,36,14>)
    n351 = xnode "Butterworth Filter"("input data"=w682, "scaled coefficients"="scaled coefficients") -> ("output data"=→"omega_p (Mavg w. f)":fxp<+/-,36,18>)  [unwired: 1 in]
  }
